vi "Demo.vi"() -> ()   [LabVIEW 2015]
uses:
  LabBASSMOD2.lvlib
panel:
  out "return type":u32
  in  "Volume":u32(slide) scale=0.0..100.0
  in  "Stop":bool
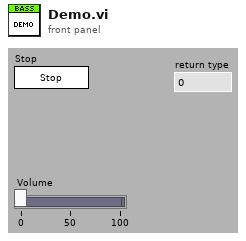
[diagram p1: front panel]
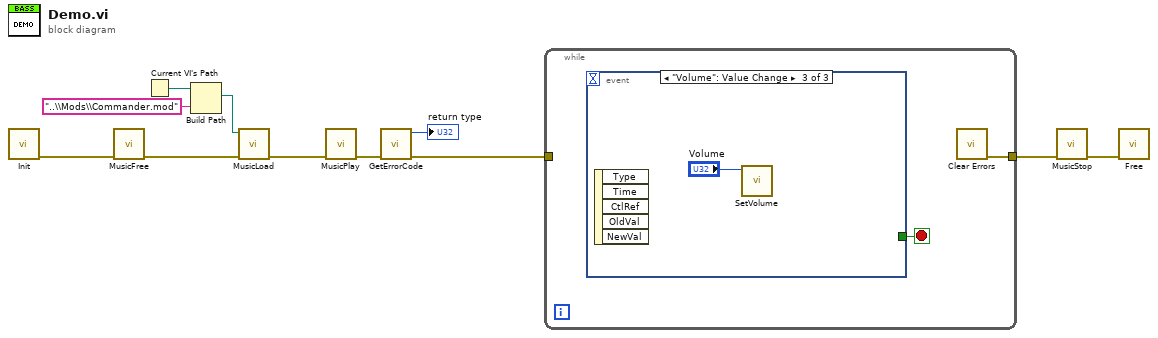
[diagram p0: block diagram]
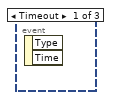
[diagram p2: hidden frame]
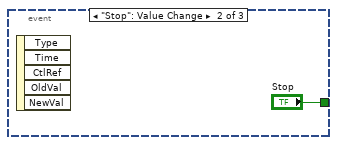
[diagram p3: hidden frame]
diagram:
  n1 = call "Init.vi"() -> ("error out"=w11:errorcluster)  [unwired: 10 in, 1 out]
  n2 = call "MusicFree.vi"("error in (no error)"=w11) -> ("error out"=w9:errorcluster)  [unwired: 10 in]
  n3 = Current VI's Path() -> (path=w3:path)
  n4 = Build Path(base path=w3, name or relative path="..\\Mods\\Commander.mod") -> (appended path=w1:path)
  n5 = call "MusicLoad.vi"("error in (no error)"=w9, "path"=w1) -> ("error out"=w8:errorcluster)  [unwired: 9 in]
  n6 = call "MusicPlay.vi"("error in (no error)"=w8) -> ("error out"=w7:errorcluster)  [unwired: 10 in]
  n7 = call "GetErrorCode.vi"("error in (no error)"=w7) -> ("error out"=w6:errorcluster, "Error Code"=→"return type":u32)  [unwired: 9 in]
  n8 = while {
    tunnel: w6 -> [_]
    tunnel: [w12] -> w4
    stop <- w13 stop-if-true
    n9 = event shown="[2] \"Volume\": Value Change" {
      selector: _ -> [_ _ _]
      dyn-events: _ -> [_ _ _]
      timeout: _ -> [_ _ _]
      tunnel: [_ "Stop" _] -> w13
      event Timeout {
        n10 = event-data() -> ()  [unwired: 1 in, 2 out]
      }
      event "Stop": Value Change {
        n11 = event-data() -> ()  [unwired: 1 in, 5 out]
      }
      event "Volume": Value Change {
        n12 = event-data() -> ()  [unwired: 1 in, 5 out]
        n13 = call "SetVolume.vi"("Volume"="Volume") -> ()  [unwired: 10 in, 1 out]
      }
    }
    n14 = call <vilib>:"Clear Errors.vi"() -> ("error out"=w12:errorcluster)  [unwired: 6 in, 1 out]
  }
  n15 = call "MusicStop.vi"("error in (no error)"=w4) -> ("error out"=w10:errorcluster)  [unwired: 10 in]
  n16 = call "Free.vi"("error in (no error)"=w10) -> ()  [unwired: 10 in, 1 out]
